vi "Get Name.vi"(11 "Object Entry in":refnum<class "Section.lvclass">) -> (2 "Section Name":refnum<class "Section Name.lvclass">, 3 "Object Entry out":refnum<class "Section.lvclass">)   [LabVIEW 2024, in "EDS.lvlib" / "Section.lvclass"]
uses:
  Section.lvclass
  Section.lvclass/Section.ctl
  Section Name/Section Name.lvclass
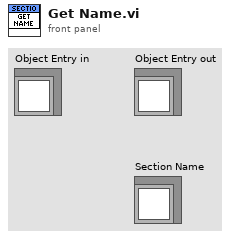
[diagram p1: front panel]
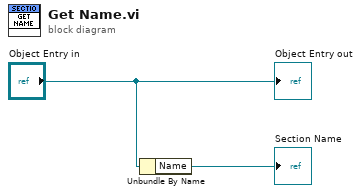
[diagram p0: block diagram]
diagram:
  n1 = Unbundle By Name("Object Entry in") -> ("Name"=→"Section Name":refnum<class "Section Name.lvclass">)
  "Object Entry out" <- "Object Entry in"
